vi "FFT1D.vi"() -> ()   [LabVIEW 2020]
doc: "This benchmark is designed to demonstrate execution performance improvement when executing FFT and IFFT operations on a GPU."
uses:
  956bade7-a26b-4376-82d1-4f43b9b25d0c.vi
  a45b64e6-426e-4566-b00d-58499d731ec9.vi
  <vilib>/Analysis/2dsp.llb/Real FFT.vi
  <vilib>/Analysis/2dsp.llb/Inverse Real FFT.vi
  2d4acfdf-3b2f-4360-8aac-546d4cc334b7.vi
  e3d6266a-341e-462f-8124-2d714a455819.vi
  <vilib>/Utility/High Resolution Relative Seconds.vi
  <vilib>/Ngene/CuLab - GPU Accelerated Toolkit/Toolkit/Low_Level/Tensor_Classes/T_Children/T1D/T1D_Children/T1D_SGL/Pull.vi
  <vilib>/Ngene/CuLab - GPU Accelerated Toolkit/Toolkit/API/Signal Processing/Transforms/CU_IFFT/T1D/CU_IFFT_T1D_C2R.vi
  <vilib>/Ngene/CuLab - GPU Accelerated Toolkit/Toolkit/API/Signal Processing/Transforms/CU_FFT/T1D/CU_FFT_T1D_R2C.vi
  <vilib>/Ngene/CuLab - GPU Accelerated Toolkit/Toolkit/Low_Level/Tensor_Classes/T_Children/T1D/T1D_Children/T1D_SGL/Push.vi
  <vilib>/Ngene/CuLab - GPU Accelerated Toolkit/Toolkit/Low_Level/Tensor_Classes/T_Children/T1D/T1D_Children/T1D_SGL/Create_Push.vi
  <vilib>/Analysis/NI_AALBase.lvlib
  <vilib>/Ngene/CuLab - GPU Accelerated Toolkit/Toolkit/CuLab.lvlib
  <vilib>/Analysis/NI_AALPro.lvlib
  <vilib>/Ngene/CuLab - GPU Accelerated Toolkit/Toolkit/Low_Level/Tensor_Classes/T_Children/T1D/T1D_Children/T1D_SGL/T1D_SGL.lvclass
panel:
  out "Improvement":dbl[](array[numeric])=[36.50360161856616, 36.185390325613305, 32.351256610011, 23.08342449593315, 18.012349103850973, 12.973898855180295, 11.137741951849097, 8.067769605828097, 5.418153632890173, 3.7918215982069228, 1.639118464616597, 0.7101025180299668, 0.38249590933755945, 0.1783960621707361] format="%.2f"
  out "Iteration":i32=9
  out "FFT_Size":i32=1024
  out "Computing on":string="CPU"
  out "GPU Model":string="NVIDIA GeForce GTX 1650 Ti"
  out "CPU Model":string="Intel(R) Core(TM) i7-10750H CPU @ 2.60GHz  "
  in  "No. of Repetitions":i32=10
  in  "FFT Size Stop (2^N)":i32=23
  in  "FFT Size Start (2^N)":i32=10
  out "FFT Sizes":i32[](array[numeric])=[8388608, 4194304, 2097152, 1048576, 524288, 262144, 131072, 65536, 32768, 16384, 8192, 4096, 2048, 1024] format="%.2p"
  out "Performance Improvement":cluster{i32[], dbl[]}(graph)={[8388608, 4194304, 2097152, 1048576, 524288, 262144, 131072, 65536, 32768, 16384, 8192, 4096, 2048, 1024], [36.50360161856616, 36.185390325613305, 32.351256610011, 23.08342449593315, 18.012349103850973, 12.973898855180295, 11.137741951849097, 8.067769605828097, 5.418153632890173, 3.7918215982069228, 1.639118464616597, 0.7101025180299668, 0.38249590933755945, 0.1783960621707361]}
  out "Execution Times":cluster{i32[], "FFT mean Exec Time":dbl[]}[](graph)=[{[8388608, 4194304, 2097152, 1048576, 524288, 262144, 131072, 65536, 32768, 16384, 8192, 4096, 2048, 1024], "FFT mean Exec Time"=[0.5604835999984061, 0.263929000000644, 0.11997139999948558, 0.04432710000037332, 0.01939929999934975, 0.00795300000027055, 0.00345269999888842, 0.0015119000017875805, 0.0006983999992371537, 0.0003060000017285347, 0.00011900000026798807, 4.850000186706893e-05, 2.359999780310318e-05, 1.089999932446517e-05]}, {[8388608, 4194304, 2097152, 1048576, 524288, 262144, 131072, 65536, 32768, 16384, 8192, 4096, 2048, 1024], "FFT mean Exec Time"=[0.015354200000729179, 0.0072938000012072735, 0.003708399999595713, 0.001920299997436814, 0.0010770000008051284, 0.0006130000001576263, 0.0003099999994446989, 0.00018739999723038636, 0.00012889999925391749, 8.069999967119657e-05, 7.259999983943999e-05, 6.829999983892776e-05, 6.170000051497482e-05, 6.10999995842576e-05]}]
  # "Overview: 1D FFT Benchmark.\nRequirements: PC with Nvidia GPU, with latest version of GPU driver and CuLab Toolkit installed.\nInstructions:\n1. Run the VI with the current benchmarking parameters.\n2. Wait for the completion of the execution. \nNote: It might take some time to perform the computations.\n3. Observe the timing and speedup results on the graphs."
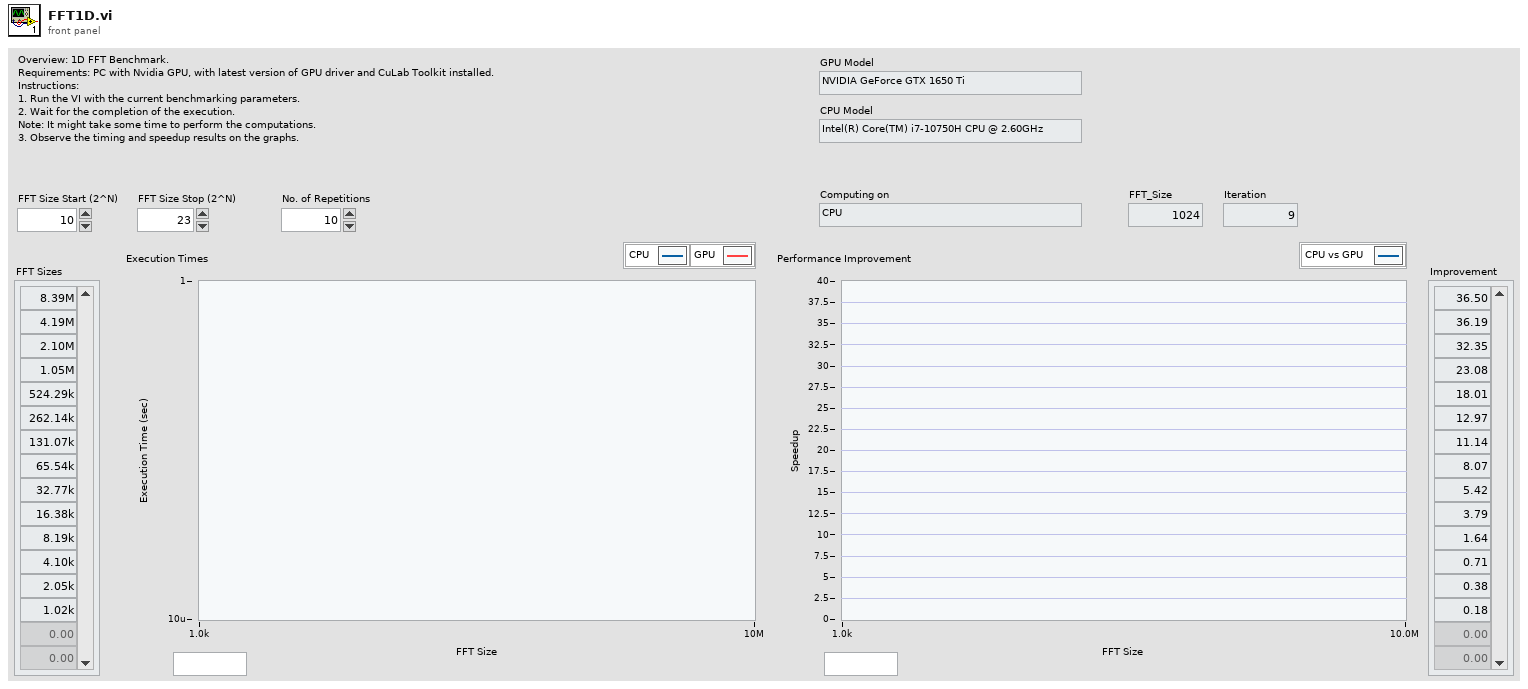
[diagram p1: front panel]
types:
  T1 = typedef "CuLab.lvlib/Properties.ctl" = cluster{"Index":i32, "Name":string}
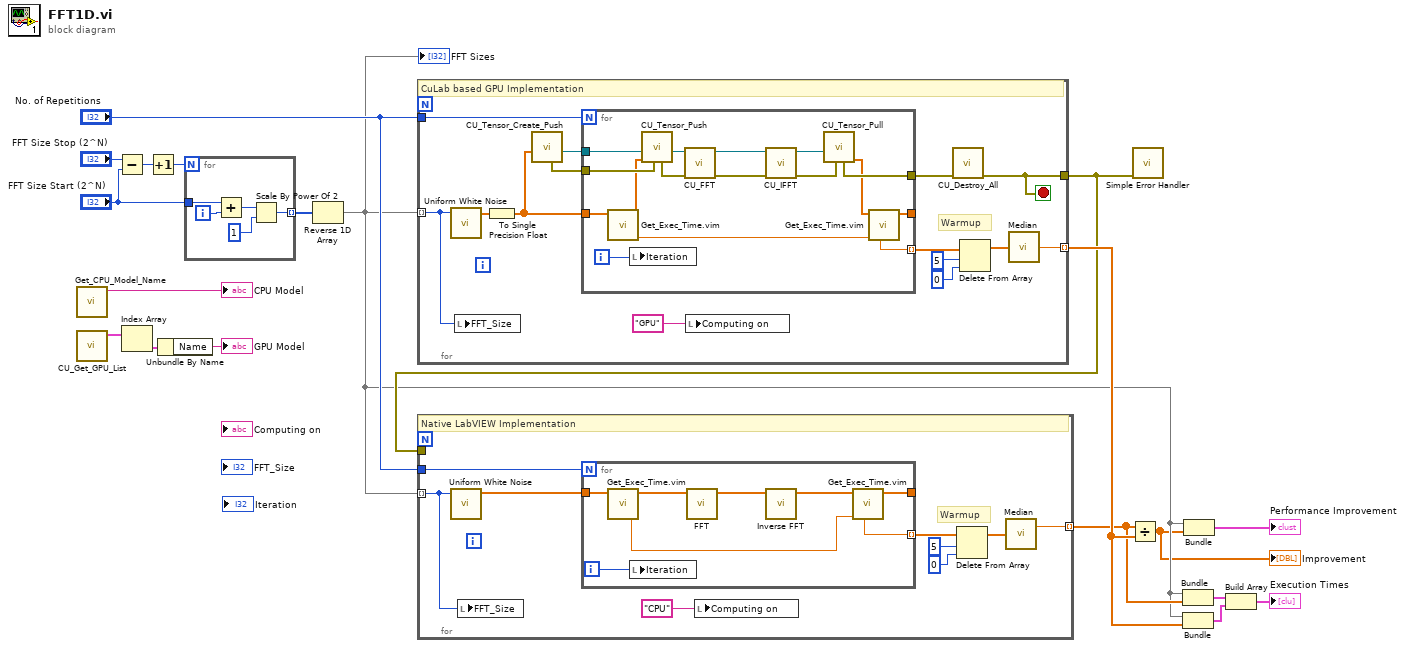
[diagram p0: block diagram]
diagram:
  n1 = call "Get_CPU_Model_Name.vi"() -> ("CPU Model"=→"CPU Model":string)  [unwired: 11 in]
  n2 = call <vilib>:"CU_Get_GPU_List.vi"() -> ("Devices"=w10:T1[])  [unwired: 10 in, 1 out]
  n3 = Subtract(x="FFT Size Stop (2^N)", y="FFT Size Start (2^N)") -> (x-y=w18:i32)
  n4 = Index Array(array=w10) -> (element=w9:T1)  [unwired: 1 in]
  n5 = Increment(x=w18) -> (x+1=w17:i32)
  n6 = Unbundle By Name(w9) -> ("Name"=→"GPU Model":string)
  n7 = for {
    N: w17 -> [_]
    tunnel: "FFT Size Start (2^N)" -> [w24]
    tunnel: [w20] -> w13 mode=indexing
    i -> [w23]
    n8 = Add(x=w24, y=w23) -> (x+y=w22:i32)
    n9 = Scale By Power Of 2(n=w22, x=1) -> (x*2^n=w20:i32)
  }
  n10 = Reverse 1D Array(array=w13) -> (reversed array=w2:i32[])
  "FFT Sizes" <- w2
  n11 = for {
    tunnel: [w27] -> w12
    tunnel: [w36] -> w14 mode=indexing
    tunnel: w2 -> [w25] mode=indexing
    tunnel: "No. of Repetitions" -> [w32]
    stop <- w27 stop-if-true
    # "Warmup"
    # "CuLab based GPU Implementation"
    n12 = call <vilib>:"Uniform White Noise.vi"("samples"=w25) -> ("uniform white noise"=w28:dbl[])  [unwired: 9 in, 1 out]
    n13 = local write "FFT_Size"(w25) -> ()
    n14 = To Single Precision Float(number=w28) -> (single precision float=w29:sgl[])
    n15 = call-poly <vilib>:"CU_Tensor_Create_Push.vi"("CPU_Data_1D_SGL"=w29) -> ("T1D_SGL out"=w38:refnum<class "T1D_SGL.lvclass">, "error out"=w37:errorcluster)  [unwired: 9 in]
    n16 = for {
      N: w32 -> [_]
      tunnel: w38 -> [w49]
      tunnel: w37 -> [w44]
      tunnel: [w43] -> w31
      tunnel: [w50] -> w30 mode=indexing
      tunnel: w29 -> [w42]
      tunnel: [w39] -> _
      i -> [w45]
      n17 = call "Get_Exec_Time.vim"("error in (no error)"=w42) -> ("T(n)"=w51:dbl, "error out"=w41:sgl[])  [unwired: 6 in, 1 out]
      n18 = local write "Iteration"(w45) -> ()
      n19 = call-poly <vilib>:"CU_Tensor_Push.vi"("error in (no error)"=w44, "CPU_Data_1D_SGL"=w41, "T1D_SGL in"=w49) -> ("T1D_SGL out"=w46:refnum<class "T1D_SGL.lvclass">, "error out"=w54:errorcluster)  [unwired: 7 in]
      n20 = call-poly <vilib>:"CU_FFT.vi"("error in"=w54, "X"=w46) -> ("error out"=w47:errorcluster, "FFT {X}"=w48:refnum<class "T1D_CSG.lvclass">)  [unwired: 8 in]
      n21 = call-poly <vilib>:"CU_IFFT.vi"("error in"=w47, "FFT {X}"=w48) -> ("error out"=w53:errorcluster, "X"=w52:refnum<class "T1D_SGL.lvclass">)  [unwired: 8 in]
      n22 = call-poly <vilib>:"CU_Tensor_Pull.vi"("error in (no error)"=w53, "T1D_SGL in"=w52) -> ("Dest out"=w40:sgl[], "error out"=w43:errorcluster)  [unwired: 7 in, 1 out]
      n23 = call "Get_Exec_Time.vim"("T(n-1)"=w51, "error in (no error)"=w40) -> ("error out"=w39:sgl[], "dT"=w50:dbl)  [unwired: 5 in, 1 out]
    }
    n24 = local write "Computing on"("GPU" ("Info")) -> ()
    n25 = call <vilib>:"CU_Destroy_All.vi"("error in"=w31) -> ("error out"=w27:errorcluster)  [unwired: 10 in]
    n26 = Delete From Array(array=w30, length=5, index=0) -> (array with subset deleted=w35:dbl[])  [unwired: 1 out]
    n27 = call <vilib>:"Median.vi"("X"=w35) -> ("median"=w36:dbl)  [unwired: 1 out]
  }
  n28 = for {
    tunnel: [w59] -> w5 mode=indexing
    tunnel: w2 -> [w55] mode=indexing
    tunnel: "No. of Repetitions" -> [w58]
    tunnel: w12 -> [_]
    # "Warmup"
    # "Native LabVIEW Implementation"
    n29 = call <vilib>:"Uniform White Noise.vi"("samples"=w55) -> ("uniform white noise"=w57:dbl[])  [unwired: 9 in, 1 out]
    n30 = local write "FFT_Size"(w55) -> ()
    n31 = for {
      N: w58 -> [_]
      tunnel: w57 -> [w70]
      tunnel: [w67] -> _
      tunnel: [w65] -> w63 mode=indexing
      i -> [w64]
      n32 = call "Get_Exec_Time.vim"("error in (no error)"=w70) -> ("T(n)"=w66:dbl, "error out"=w68:dbl[])  [unwired: 6 in, 1 out]
      n33 = local write "Iteration"(w64) -> ()
      n34 = call-poly <vilib>:"FFT.vi"("X"=w68) -> ("FFT {X}"=w71:cdb[])  [unwired: 9 in, 1 out]
      n35 = call-poly <vilib>:"Inverse FFT.vi"("FFT {X}"=w71) -> ("X"=w69:dbl[])  [unwired: 9 in, 1 out]
      n36 = call "Get_Exec_Time.vim"("T(n-1)"=w66, "error in (no error)"=w69) -> ("error out"=w67:dbl[], "dT"=w65:dbl)  [unwired: 5 in, 1 out]
    }
    n37 = local write "Computing on"("CPU" ("Info")) -> ()
    n38 = Delete From Array(array=w63, length=5, index=0) -> (array with subset deleted=w60:dbl[])  [unwired: 1 out]
    n39 = call <vilib>:"Median.vi"("X"=w60) -> ("median"=w59:dbl)  [unwired: 1 out]
  }
  n40 = Divide(x=w5, y=w14) -> (x/y=w1:dbl[])
  "Improvement" <- w1
  n41 = call <vilib>:"Simple Error Handler.vi"("error in (no error)"=w12) -> ()  [unwired: 4 in, 5 out]
  n42 = Bundle(w2, w5) -> (w7:cluster{i32[], dbl[]})  [unwired: 1 in]
  n43 = Bundle(w2, w14) -> (w6:cluster{i32[], dbl[]})  [unwired: 1 in]
  n44 = Bundle(w2, w1) -> (→"Performance Improvement":cluster{i32[], dbl[]})  [unwired: 1 in]
  n45 = Build Array(w7, w6) -> (→"Execution Times":cluster{i32[], dbl[]}[])
